vi "Configure Output.vi"(0 "VISA resource name":refnum<visa-resource-name>, 1 "Manual Range(0.00)":dbl format="%.2f", 7 "Function(0:Voltage)":u16(ring) items=["Voltage", "Current"], 9 "Enable Output (T: Enable)":bool=TRUE, 11 "error in (no error)":errorcluster, 12 "Unit(V)":u16(ring) items=["V", "mV", "kV", "A", "mA"]) -> (4 "VISA resource name out":refnum<visa-resource-name>, 15 "error out":errorcluster)   [LabVIEW 2013, in "Keithley 2200 Series.lvlib"]
doc: "Configure voltage or current value.\nSelect the output on/off and then set the Voltage or current value as per the selection of the voltage and current."
uses:
  Keithley 2200 Series.lvlib
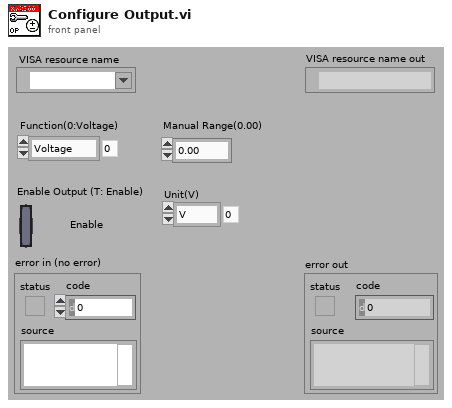
[diagram p1: front panel]
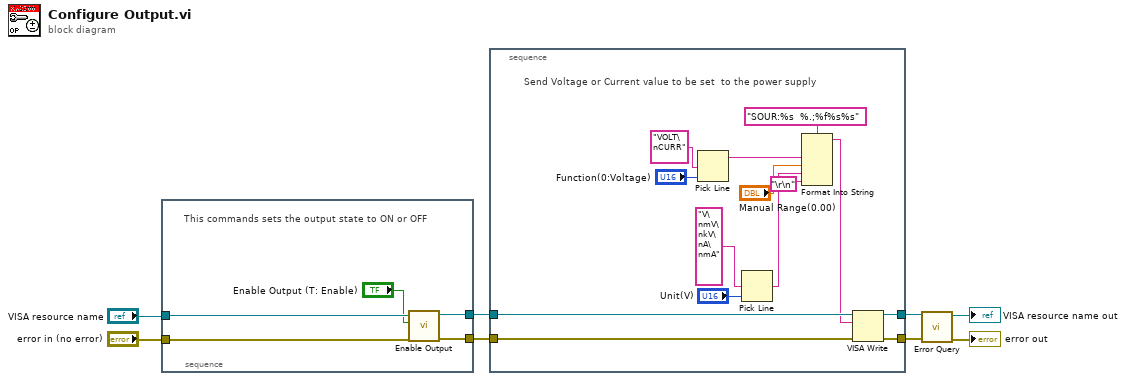
[diagram p0: block diagram]
diagram:
  n1 = stacked-sequence {
    tunnel: "VISA resource name" -> [w13]
    tunnel: "error in (no error)" -> [w12]
    tunnel: [w11] -> w4
    tunnel: [w10] -> w3
    frame #0 {
      # "This commands sets the output state to ON or OFF"
      n2 = call "Enable Output.vi"("error in (no error)"=w12, "Enable Output (T: Enable)"="Enable Output (T: Enable)", "VISA resource name"=w13) -> ("error out"=w10:errorcluster, "VISA resource name out"=w11:refnum<visa-resource-name>)  [unwired: 7 out]
    }
  }
  n3 = stacked-sequence {
    tunnel: [w27] -> w8
    tunnel: [w26] -> w7
    tunnel: w4 -> [w19]
    tunnel: w3 -> [w18]
    frame #0 {
      # "Send Voltage or Current value to be set  to the power supply"
      n4 = Pick Line(multi-line string="VOLT\nCURR" ("format string"), line index="Function(0:Voltage)") -> (output string=w20:string)  [unwired: 1 out]
      n5 = Pick Line(multi-line string="V\nmV\nkV\nA\nmA", line index="Unit(V)") -> (output string=w21:string)  [unwired: 1 out]
      n6 = Format Into String(format string="SOUR:%s  %.;%f%s%s", w20, "Manual Range(0.00)", w21, "\r\n" ("End of Line Constant")) -> (resulting string=w14:string)  [unwired: 2 in, 1 out]
      n7 = VISA Write(VISA resource name=w19, write buffer=w14, error in (no error)=w18) -> (VISA resource name out=w27:refnum<visa-resource-name>, error out=w26:errorcluster)  [unwired: 1 out]
    }
  }
  n8 = call "Error Query.vi"("error in (no error)"=w7, "VISA resource name"=w8) -> ("error out"=→"error out":errorcluster, "VISA resource name out"=→"VISA resource name out":refnum<visa-resource-name>)  [unwired: 8 out]
